vi "WaitPassTacticCheckStateChange.vi"(6 "states in":T1, 8 "error in (no error)":errorcluster, 9 "Robot in":refnum<class "Robot.lvclass">, 10 "Game":refnum<class "Game.lvclass">, 11 "WaitPassTactic in":refnum<class "WaitPassTactic.lvclass">) -> (0 "error out":errorcluster, 2 "states out":T1, 3 "WaitPassTactic out":refnum<class "WaitPassTactic.lvclass">)   [LabVIEW 2024, in "WaitPassTactic.lvclass"]
uses:
  WaitPassTactic.lvclass
  Game_class/Game.lvclass
  Robot_class/Robot.lvclass
  C:/Users/moise/Documents/GitHub/SSL_AI/Object_class/Object.lvclass
  Controls/StatesPass.ctl
  Object_class/Object.lvclass/Object.ctl
  Robot_class/Robot.lvclass/Robot.ctl
  Robot_class/Read id.vi
  Object_class/Read position(x,y).vi
  Robot_class/Read Zone.vi
  Robot_class/Read orientation.vi
  Robot_class/Read dest_orientation.vi
  Zone_class/Zone.lvclass
  Utilities_class/Utilities.lvclass
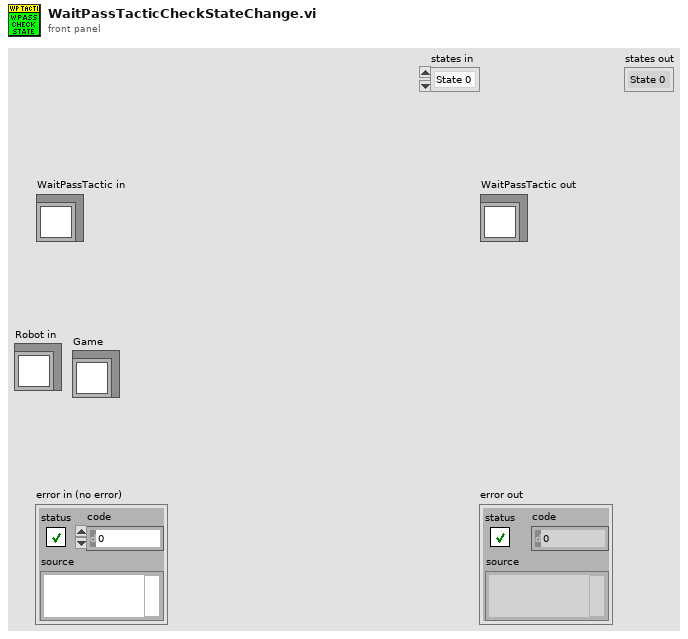
[diagram p1: front panel]
types:
  T1 = typedef "StatesPass.ctl" = enum16{"State 0", "State 1", "State 2", "State 3", "Exit"}
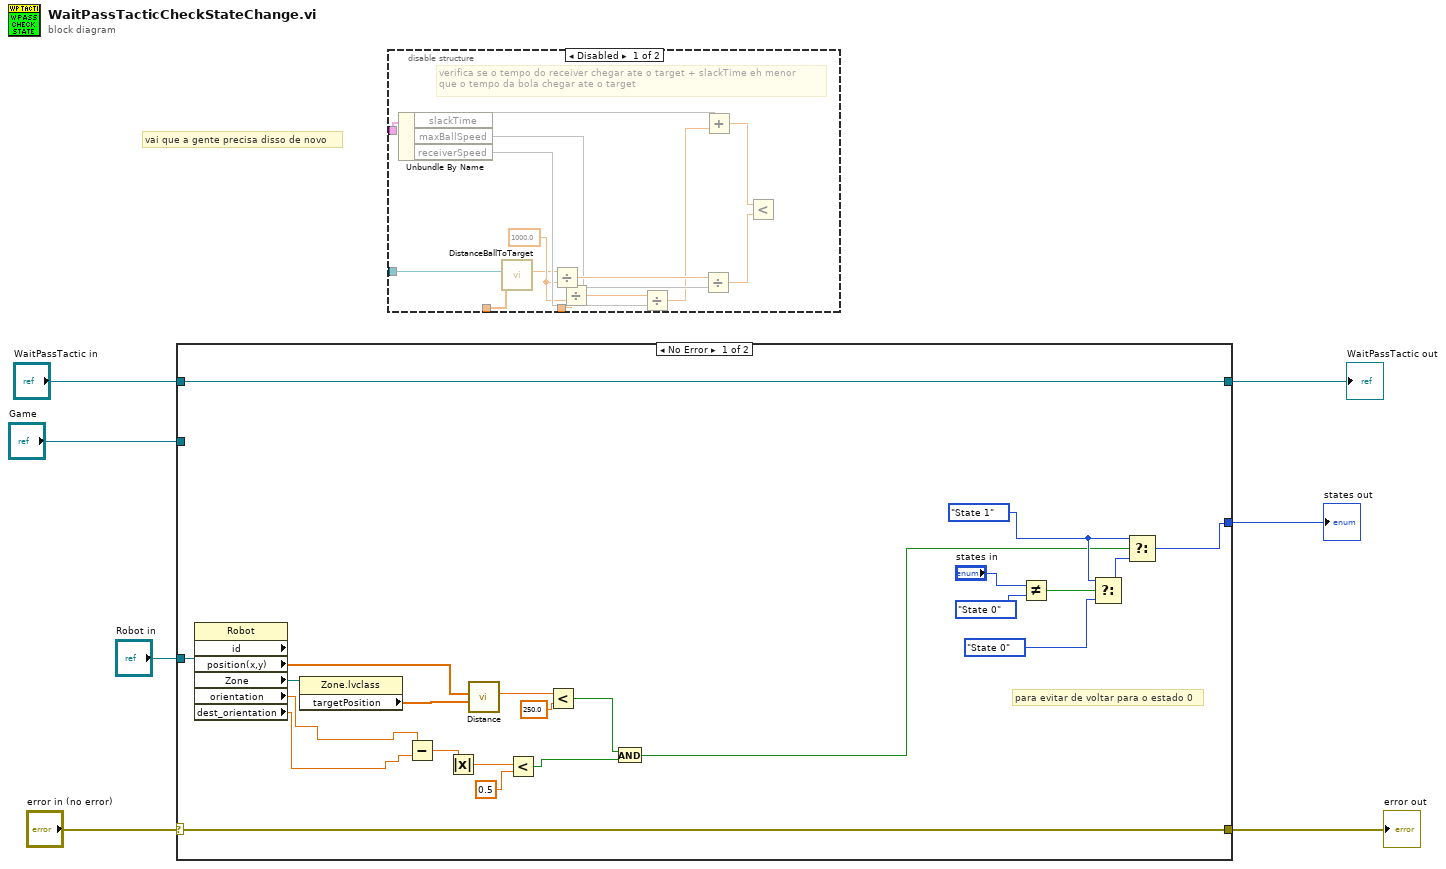
[diagram p0: block diagram]
diagram:
  # "vai que a gente precisa disso de novo"
  n1 = case shown="No Error" "error in (no error)" {
    selector: "error in (no error)" -> [w30 w32]
    tunnel: [w30 w32] -> w6
    tunnel: [w29 w31] -> w4
    tunnel: "WaitPassTactic in" -> [w29 w31]
    tunnel: "Game" -> [_ _]
    tunnel: "Robot in" -> [w28 _]
    tunnel: [w8 _] -> w1
    frame No Error {
      w17 = StatesPass."State 1" ("y")
      # "para evitar de voltar para o estado 0"
      n2 = property class="Robot" props=["id", "position(x,y)", "Zone", "orientation", "dest_orientation"](reference=w28) -> ("position(x,y)"=w26:dbl[], "Zone"=w27:refnum<class "Zone.lvclass">, "orientation"=w14:dbl, "dest_orientation"=w13:dbl)  [unwired: 1 in, 3 out]
      n3 = property class="Zone.lvclass"(reference=w27) -> ("targetPosition"=w19:dbl[])  [unwired: 1 in, 2 out]
      n4 = Subtract(x=w14, y=w13) -> (x-y=w12:dbl)
      n5 = Absolute Value(x=w12) -> (abs(x)=w11:dbl)
      n6 = call "Distance.vi"("P1"=w19, "P2"=w26) -> ("Distance"=w18:dbl)  [unwired: 7 in, 2 out]
      n7 = Less?(x=w11, y=0.5) -> (x < y?=w9:bool)
      n8 = Less?(x=w18, y=250.0) -> (x < y?=w16:bool)
      n9 = And(x=w16, y=w9) -> (x .and. y?=w15:bool)
      n10 = Not Equal?(x="states in", y=StatesPass."State 0") -> (x != y?=w23:bool)
      n11 = Select(t=w17, s=w23, f=StatesPass."State 0") -> (s? t:f=w22:T1)
      n12 = Select(t=w17, s=w15, f=w22) -> (s? t:f=w8:T1)
    }
    frame Error {
    }
  }
  "error out" <- w6
  "WaitPassTactic out" <- w4
  "states out" <- w1
  n13 = disable-structure shown="Disabled" {
    disable-tunnel: _ -> [w46 _]
    disable-tunnel: _ -> [w45 _]
    disable-tunnel: _ -> [w34 _]
    disable-tunnel: _ -> [w33 _]
    frame Disabled {
      w36 = 1000.0 ("y")
      # "verifica se o tempo do receiver chegar ate o target + slackTime eh menor \nque o tempo da bola chegar ate o target"
      n14 = Unbundle By Name(w46) -> ("slackTime"=w40, "maxBallSpeed"=w41, "receiverSpeed"=w43)
      n15 = call "DistanceBallToTarget.vi"("Target"=w45, "Ball"=w34) -> ("Distance Ball To Target"=w35:dbl)  [unwired: 7 in, 2 out]
      n16 = Divide(x=w35, y=w36) -> (x/y=w42:dbl)
      n17 = Divide(x=w33, y=w36) -> (x/y=w44:dbl)
      n18 = Divide(x=w44, y=w43) -> (x/y=w39:dbl)
      n19 = Divide(x=w42, y=w41) -> (x/y=w37:dbl)
      n20 = Add(x=w40, y=w39) -> (x+y=w38:dbl)
      n21 = Less?(x=w38, y=w37) -> ()  [unwired: 1 out]
    }
    frame Enabled {
    }
  }
